vi "CRYProbe Value.vi"() -> ()   [LabVIEW 2013]
panel:
  out "Source Step":string caption="aa"
  in  "Name":string
  out "Z":string
  out "Z":dbl format="%#_6p"
  in  "Number":i32
  in  "Close?":bool
  in  "Update?":bool
  out "Y":string
  out "X":string
  out "Y":dbl format="%#_6p"
  out "X":dbl format="%#_6p"
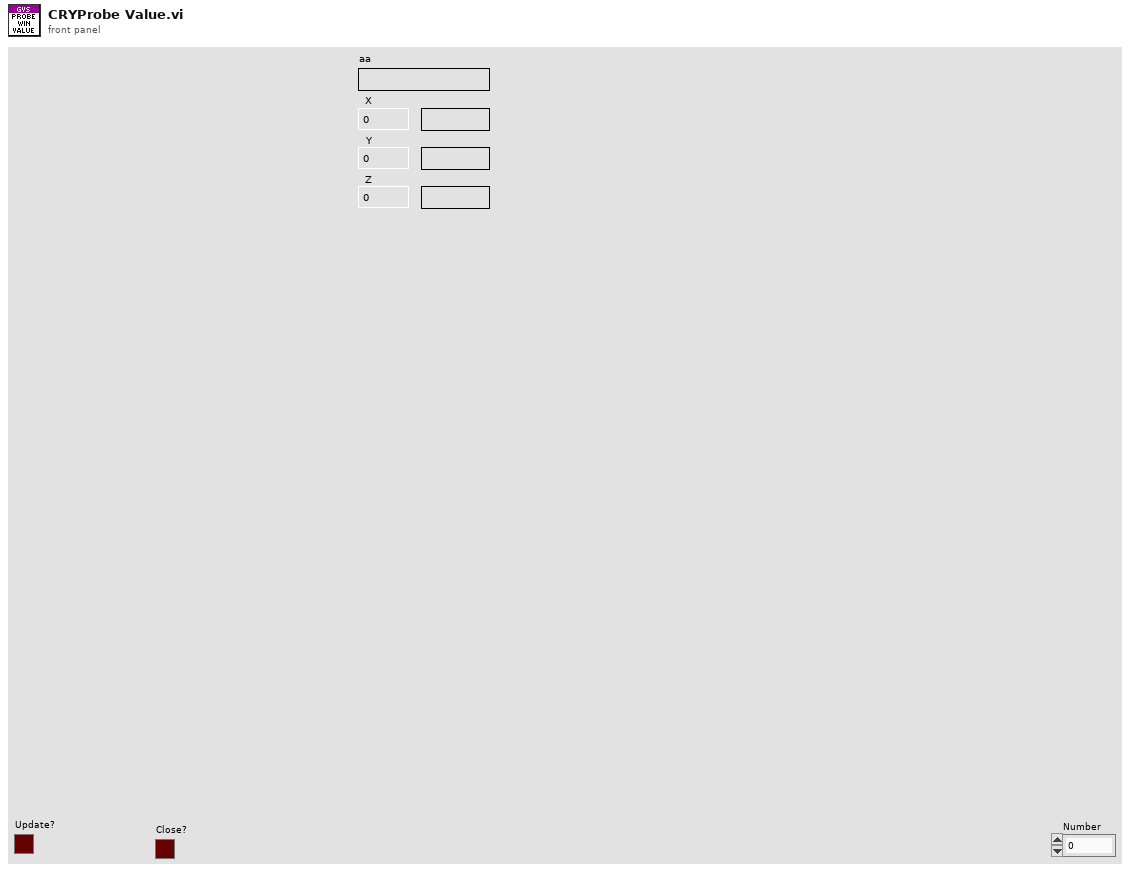
[diagram p1: front panel]
types:
  T1 = typedef "CRYData Cluster.ctl" = cluster{"Name":string, "Curve":cluster{"x":dbl, "y":dbl, "z":dbl}[], "X data":u16, "Y data":u16, "Z data":u16, "X axis":u16, "Y axis":u16, "Z axis":u16, "X unit":string, "Y unit":string, "Z unit":string, "X dB ref":dbl, "Y dB ref":dbl, "Z dB ref":dbl, "single val":bool, "protected":bool, "display X":bool, "display Y":bool, "display Z":bool, "Test Info":string, "Step No.":i32, "Plot Settings":cluster{"Color":u32, "Interpolation":u8, "Point Style":u8, "Line Style":u8, "Point Color":u32, "Line Width":u8, "Bar Plot Style":u8, "Fill To":i16}, "AutoProtect":bool}
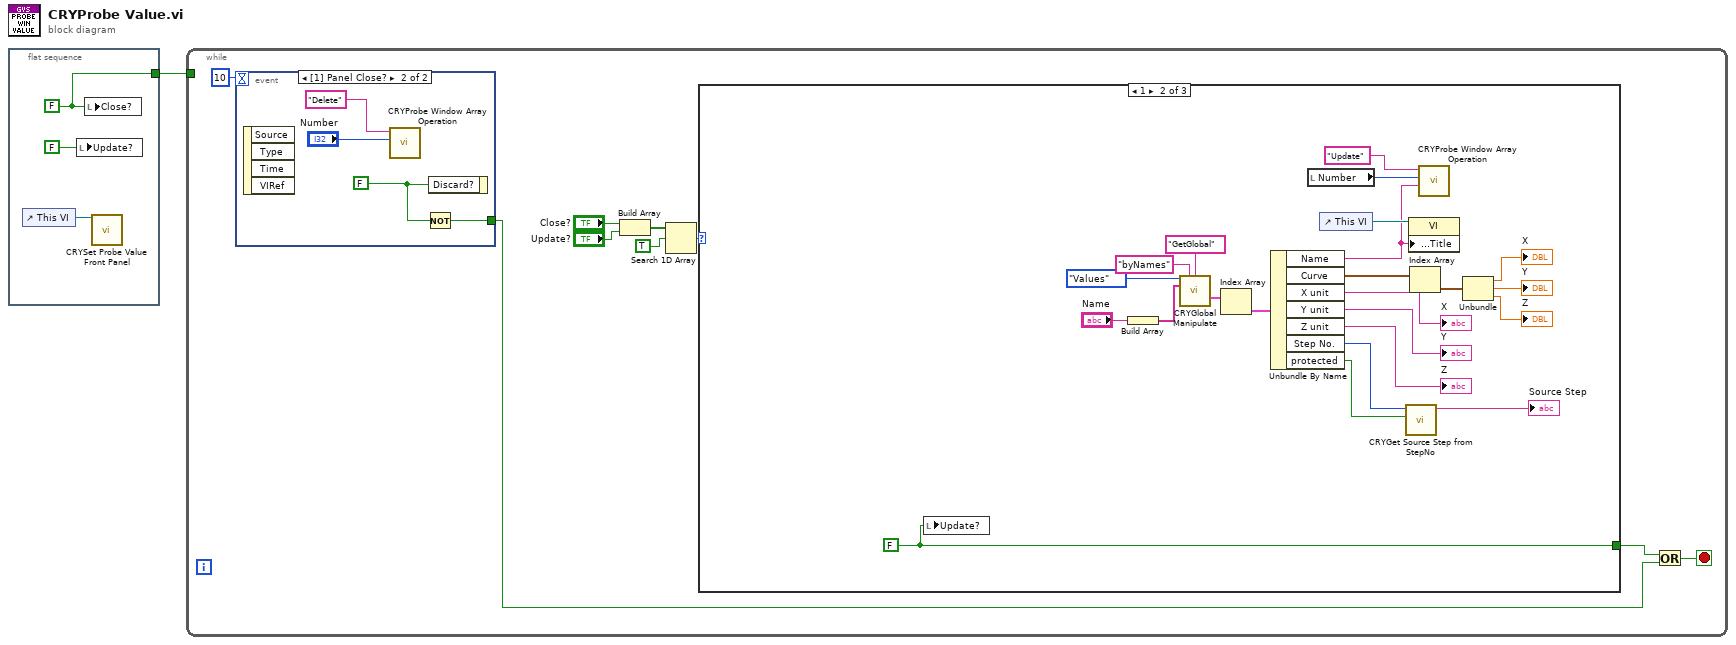
[diagram p0: block diagram]
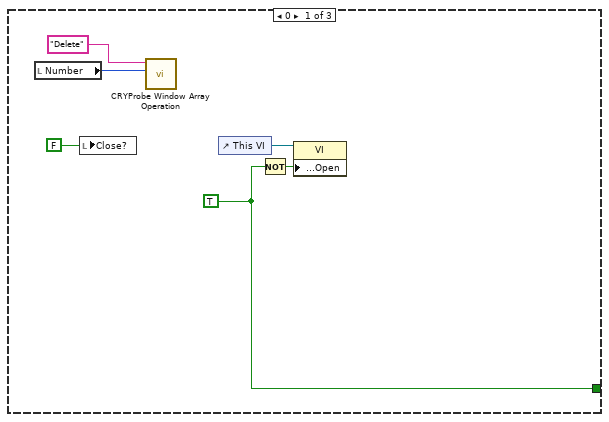
[diagram p2: hidden frame]
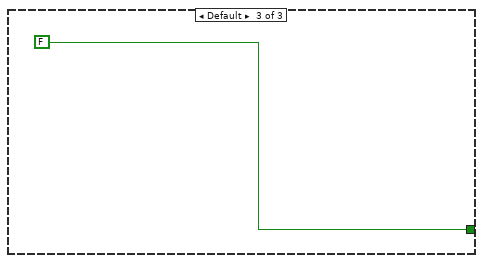
[diagram p3: hidden frame]
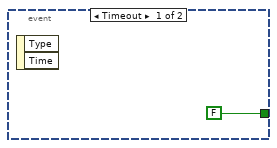
[diagram p4: hidden frame]
diagram:
  n1 = flat-sequence {
    tunnel: [w3] -> w1
    frame #0 {
      w3 = FALSE ("Close?")
      n2 = control-ref of="This VI"() -> (w2:refnum<vi>)
      n3 = local write "Update?"(FALSE ("Close?")) -> ()
      n4 = local write "Close?"(w3) -> ()
      n5 = call "CRYSet Probe Value Front Panel.vi"("Vi Ref"=w2) -> ()  [unwired: 11 in]
    }
  }
  n6 = while {
    tunnel: w1 -> [_]
    stop <- w5 stop-if-true
    n7 = event shown="[1] Panel Close?" {
      selector: _ -> [_ _]
      dyn-events: _ -> [_ _]
      timeout: 10 -> [_ _]
      tunnel: [FALSE ("Discard?") w47] -> w6
      event Timeout {
        n8 = event-data() -> ()  [unwired: 3 out]
      }
      event Panel Close? {
        w48 = FALSE ("Discard?")
        n9 = event-data() -> ()  [unwired: 5 out]
        n10 = call "CRYProbe Window Array Operation.vi"("Number"="Number", "sAction"="Delete") -> ()  [unwired: 1 in, 9 out]
        n11 = Not(x=w48) -> (.not. x?=w47:bool)
        n12 = event-data("Discard?"=w48) -> ()  [unwired: 1 in, 1 out]
      }
    }
    n13 = Build Array("Close?", "Update?") -> (w9:bool[])
    n14 = Search 1D Array(1D array=w9, element=TRUE) -> (index of element=w10:i32)  [unwired: 1 out]
    n15 = case shown="1" w10 {
      tunnel: [w16 w42 FALSE ("Close?")] -> w7
      frame 0 {
        w16 = TRUE ("Discard?")
        n16 = local read "Number"() -> (w15:i32)
        n17 = local write "Close?"(FALSE ("Close?")) -> ()
        n18 = call "CRYProbe Window Array Operation.vi"("Number"=w15, "sAction"="Delete") -> ()  [unwired: 1 in, 9 out]
        n19 = control-ref of="This VI"() -> (w17:refnum<vi>)
        n20 = Not(x=w16) -> (.not. x?=w18:bool)
        n21 = property class="VI"(reference=w17, "Front Panel.Open"=w18) -> ()  [unwired: 1 in, 2 out]
      }
      frame 1 {
        w42 = FALSE ("Close?")
        n22 = local write "Update?"(w42) -> ()
        n23 = Build Array("Name") -> (w20:string[])
        n24 = call "CRYGlobal Manipulate.vi"("Type"=enum16{"Curves", "Values", "Results", "WFM"}."Values", "sOption"="byNames", "sAction"="GetGlobal", "sData"=w20) -> ("Values Out"=w25:T1[])  [unwired: 5 in, 6 out]
        n25 = Index Array(array=w25) -> (element=w26:T1)  [unwired: 1 in]
        n26 = Unbundle By Name(w26) -> ("Name"=w32:string, "Curve"=w38:cluster{"x":dbl, "y":dbl, "z":dbl}[], "X unit"=→"X":string, "Y unit"=→"Y":string, "Z unit"=→"Z":string, "Step No."=w29:i32, "protected"=w28:bool)
        n27 = local read "Number"() -> (w31:i32)
        n28 = control-ref of="This VI"() -> (w35:refnum<vi>)
        n29 = call "CRYGet Source Step from StepNo.vi"("Protect?"=w28, "Step No."=w29) -> ("StepName"=→"Source Step":string)  [unwired: 9 in]
        n30 = property class="VI"(reference=w35, "Front Panel.Title"=w32) -> ()  [unwired: 1 in, 2 out]
        n31 = Index Array(array=w38) -> (element=w39:cluster{"x":dbl, "y":dbl, "z":dbl})  [unwired: 1 in]
        n32 = call "CRYProbe Window Array Operation.vi"("Name"=w32, "Number"=w31, "sAction"="Update") -> ()  [unwired: 9 out]
        n33 = Unbundle(w39) -> ("x"=→"X":dbl, "y"=→"Y":dbl, "z"=→"Z":dbl)
      }
      frame Default {
      }
    }
    n34 = Or(x=w7, y=w6) -> (x .or. y?=w5:bool)
  }
